vi "Main.vi"() -> ()   [LabVIEW 2022 SP3]
doc: "Use this template to build a simple state machine design pattern. Each state executes code and determines which state to transition to."
uses:
  controls/State.ctl
  <instrlib>/Vision Research Phantom Series Labview Driver/_Type Defs/PHCon IMRANGE.ctl
  <instrlib>/Vision Research Phantom Series Labview Driver/_Type Defs/PhFile InfName.ctl
  <instrlib>/Vision Research Phantom Series Labview Driver/_Type Defs/PhInt PhProcessImage Selectors.ctl
  <instrlib>/Vision Research Phantom Series Labview Driver/_Type Defs/PhInt REDUCE16TO8PARAMS.ctl
  Global 3.vi
  Global 2.vi
  Global 1.vi
  <instrlib>/Vision Research Phantom Series Labview Driver/VRI.lvlib
panel:
  in  "Weave Net":bool
  in  "Step (mm)":dbl=300.0 format="%#_13g"
  in  "Line No 2":i16=100 caption="No. of Rows"
  in  "Row spacing (um)":dbl=100.0 format="%#_13g"
  in  "Direction 2":enum16{"Y to X", "X to Y"}(ring)
  in  "Stall (s)":i16=1
  in  "Row width (mm)":dbl=60.0 format="%#_13g"
  in  "Start Pos":dbl[](array[numeric])=[-30.0, -30.0] caption="Start Point"
  in  "PtP Motion":bool
  out "XY Graph":cluster{"X":dbl, "Y":dbl}[](graph)
  out "Preview":picture
  in  "Stack No":i16=10
  in  "Direction":enum16{"Y to X", "X to Y"}(ring)
  in  "MinJT":dbl=0.02 format="%#_13g"
  in  "MaxJT":dbl=0.02 format="%#_13g"
  in  "Length (mm)":dbl=60.0 format="%#_13g"
  in  "Spacing (um)":dbl=100.0 format="%#_13g"
  in  "Line No":i16=100
  in  "Acc. (mm/s2)":dbl=1500.0 format="%#_13g"
  in  "Vel (mm/s)":dbl=300.0 format="%#_13g"
  in  "Start Point":dbl[](array[numeric])=[-30.0, -30.0]
  in  "OffsetNo":i16=20
  in  "Offsets (um,um)":dbl[](array[numeric])=[100.0, 100.0] format="%#_13g"
  in  "Repeat No":i16=1
  in  "Acc (mm/s2)":dbl=150.0 format="%#_13g"
  in  "Vel (mm/s)":dbl=70.0 format="%#_13g"
  in  "Traj file":string=".trj"
  in  "Start Position":dbl[](array[numeric])=[-30.0, -30.0] format="%#_13g"
  in  "Target":dbl[](array[numeric])=[50.0, -50.0] format="%#_13g"
  in  "Abort Current Motion":bool
  in  "Movement of Parallel Stacking":bool
  in  "Movement of Parallel Wave":bool
  in  "Move to Target":bool
  in  "Move Along Trajectory with an Offset":bool
  in  "Move Along Trajectory":bool
  in  "Disable Stage":bool
  in  "Homing Stage":bool
  in  "Exit":bool
  # "NFES CONTROL PANEL"
  # "Camera Vision"
  # "Needle position monitor"
  # "Move to Target"
  # "Trajectory Motion"
  # "Wave Motion"
  # "Point-to-Point Motion"
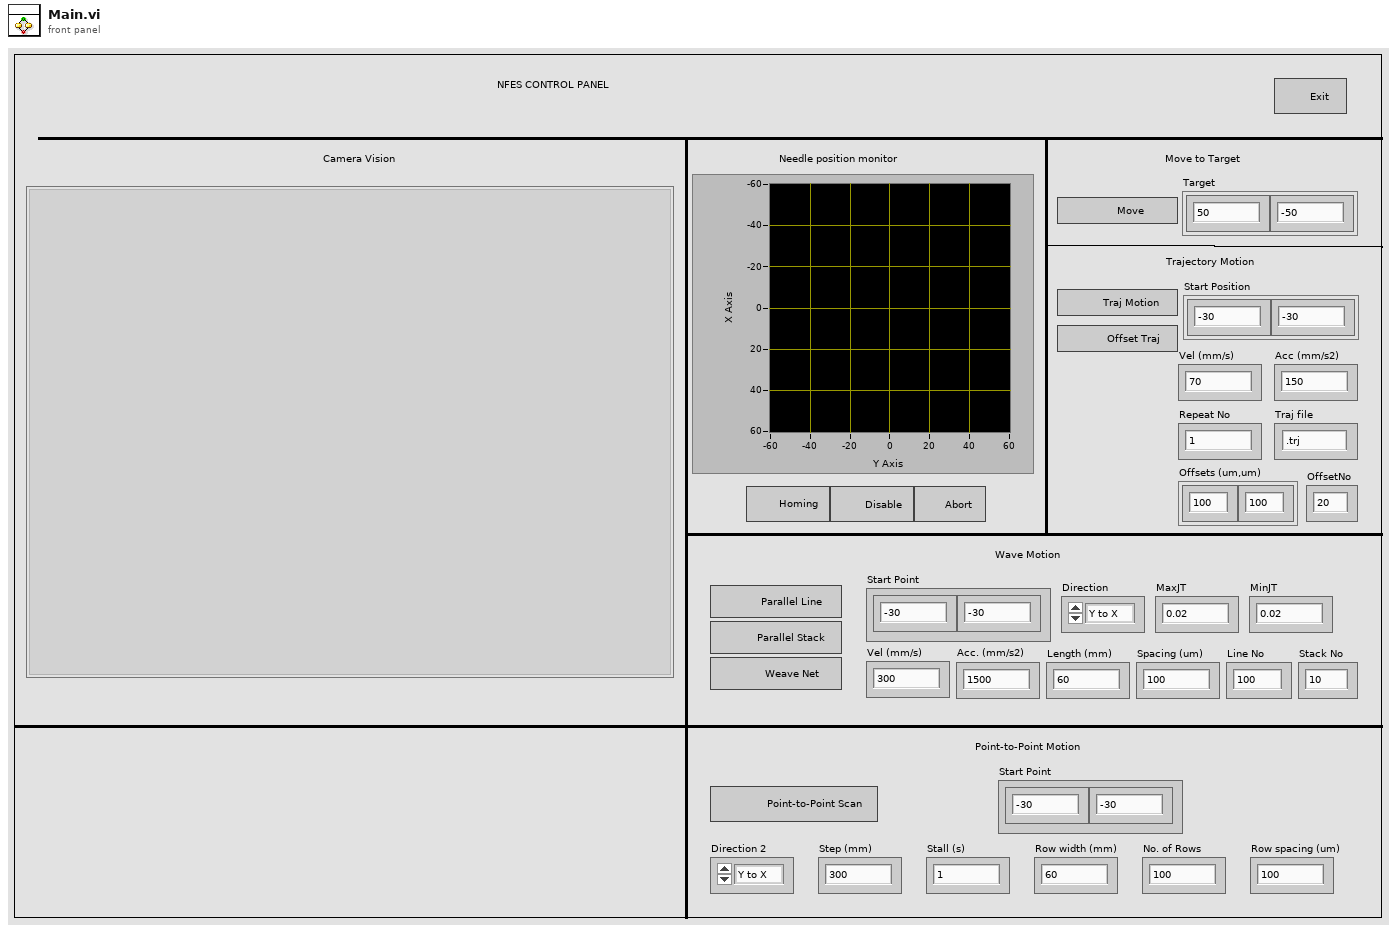
[diagram p1: front panel]
types:
  T1 = typedef "State.ctl" = enum16{"Initialize", "Wait for Event", "Homing", "Disable", "Move", "Trajectory", "Trajoffset", "ParaWave", "ParaStack", "NetWeaving", "PtPMove", "Abort", "Exit"}
  T2 = typedef "VRI.lvlib/PhInt REDUCE16TO8PARAMS.ctl" = cluster{"fGain16_8":dbl}
  T3 = typedef "VRI.lvlib/PhInt PhProcessImage Selectors.ctl" = u16
  T4 = typedef "VRI.lvlib/PhFile InfName.ctl" = u32
  T5 = typedef "VRI.lvlib/PHCon IMRANGE.ctl" = cluster{"First":i32, "Cnt":u32}
  T6 = typedef "VRI.lvlib/PhInt IH.ctl" = cluster{"biSize":u32, "biWidth":i32, "biHeight":i32, "biPlanes":u16, "biBitCount":u16, "biCompresssion":u32, "biSizeImage":u32, "biXPelsPerMeter":i32, "biYPelsPerMeter":i32, "biClrUsed":u32, "biClrImportant":u32, "BlackLevel":i32, "WhiteLevel":i32}
  T7 = typedef "VRI.lvlib/BITMAPINFOHEADER.ctl" = cluster{"biSize":u32, "biWidth":i32, "biHeight":i32, "biPlanes":u16, "biBitCount":u16, "biCompression":u32, "biSizeImage":u32, "biXPelsPerMeter":i32, "biYPelsPerMeter":i32, "biClrUsed":u32, "biClrImportant":u32}
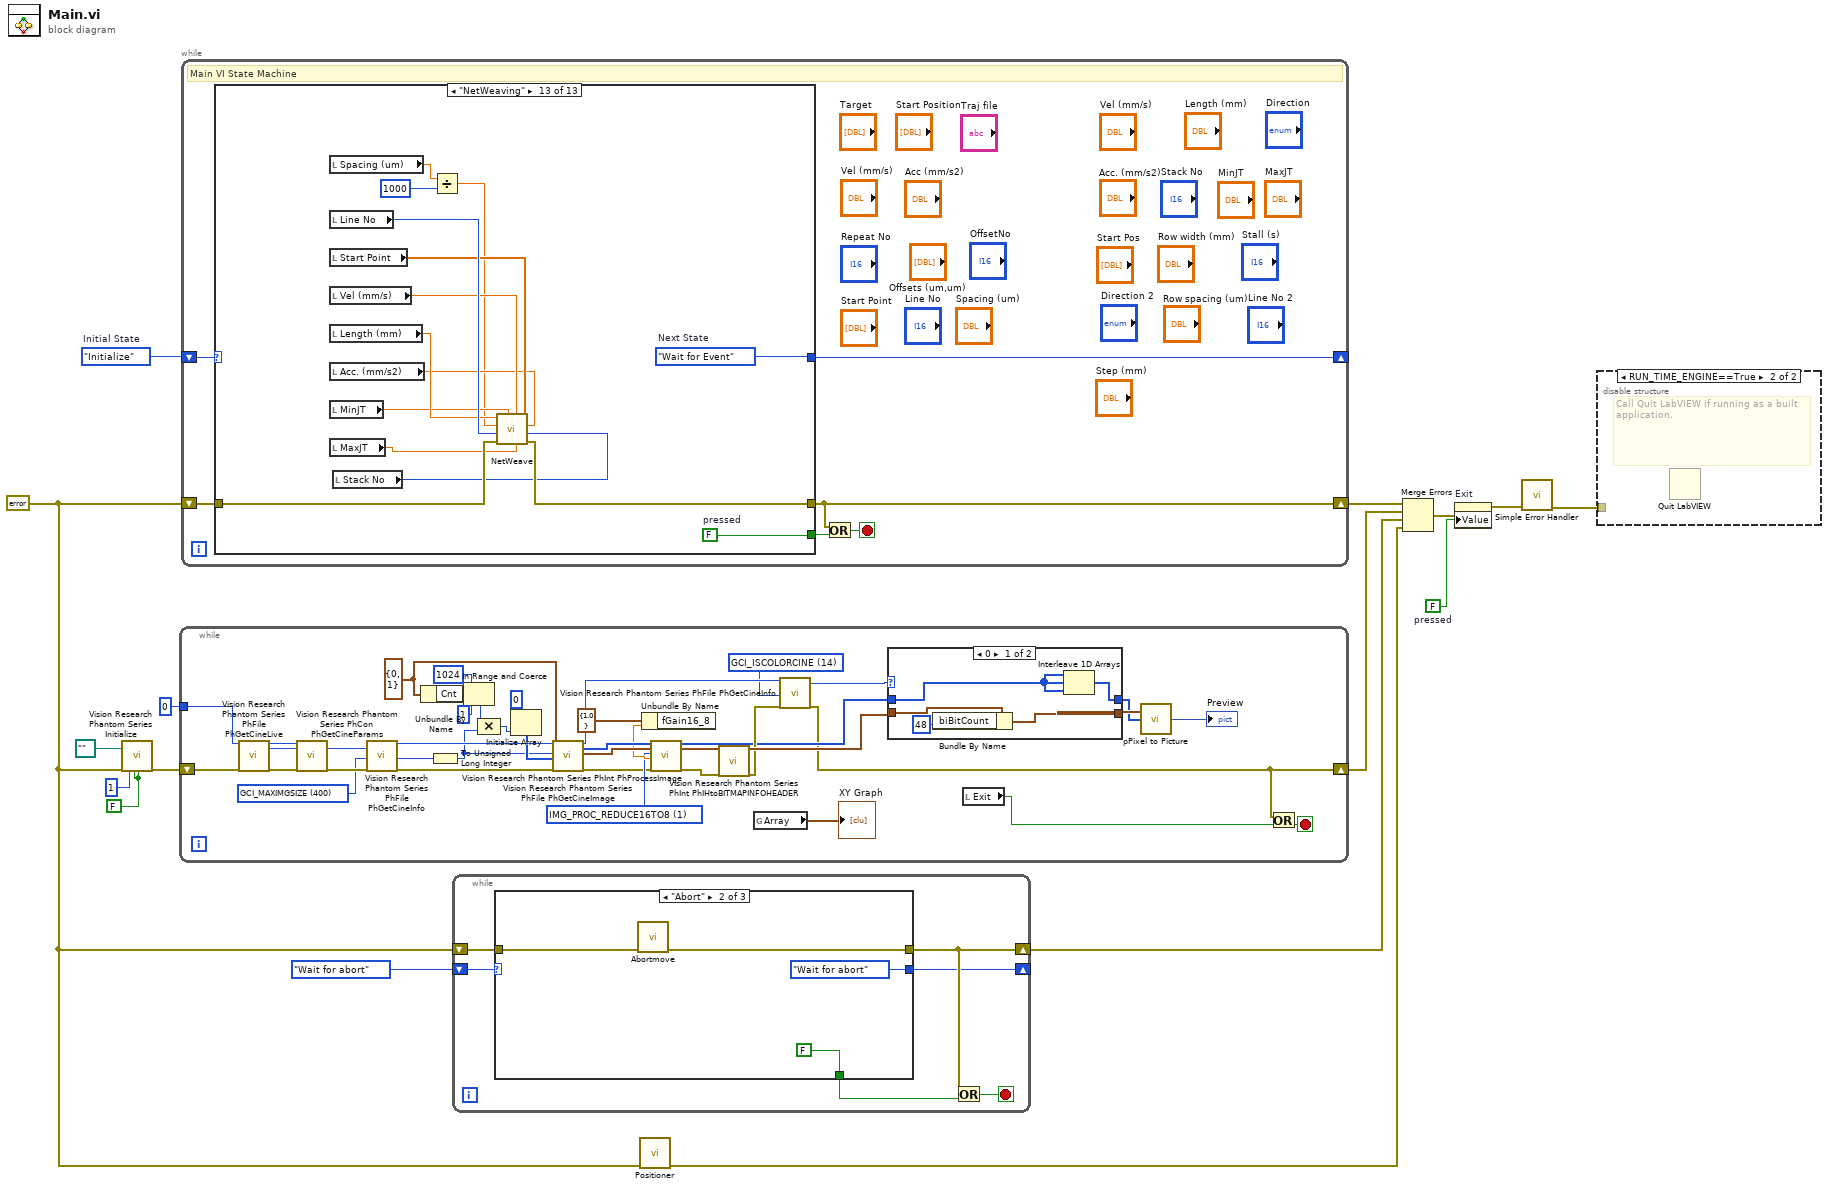
[diagram p0: block diagram]
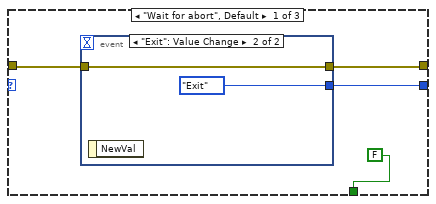
[diagram p2: hidden frame]
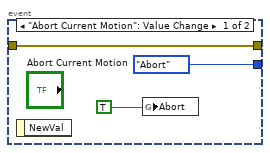
[diagram p3: hidden frame]
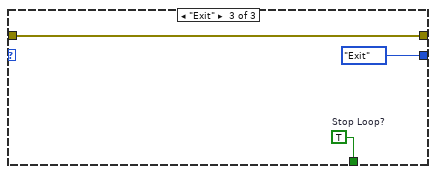
[diagram p4: hidden frame]
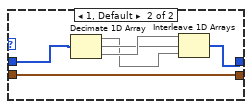
[diagram p5: hidden frame]
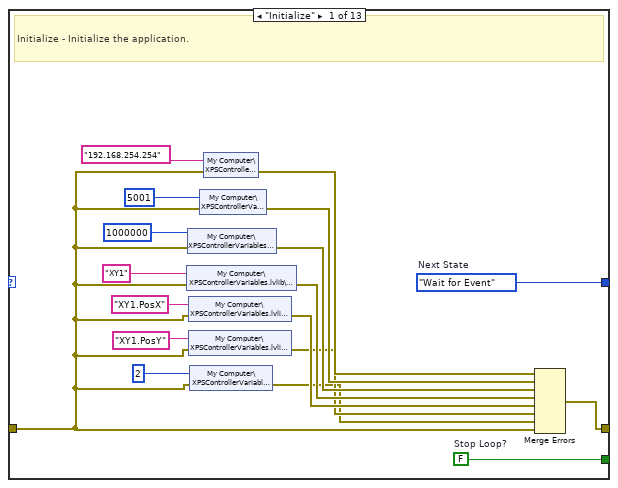
[diagram p7: hidden frame]
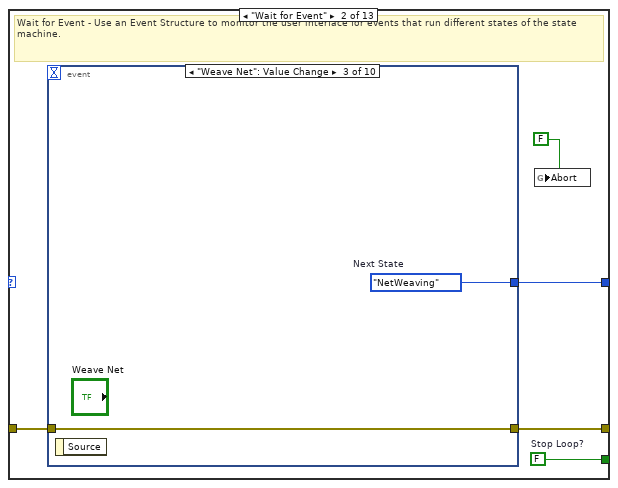
[diagram p8: hidden frame]
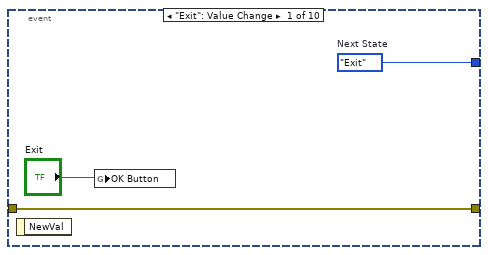
[diagram p9: hidden frame]
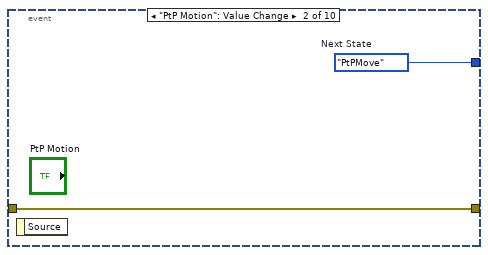
[diagram p10: hidden frame]
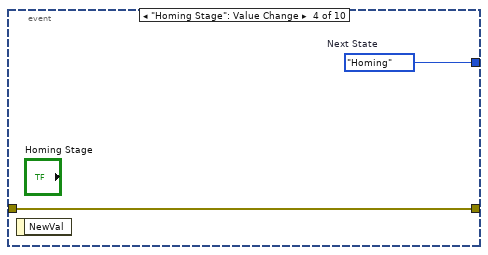
[diagram p11: hidden frame]
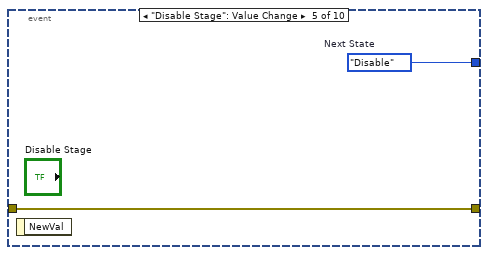
[diagram p12: hidden frame]
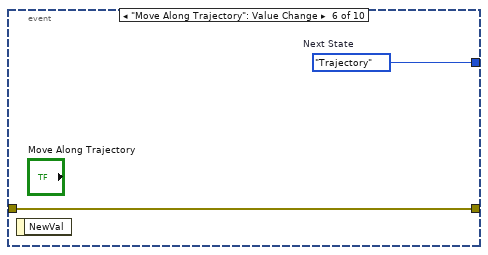
[diagram p13: hidden frame]
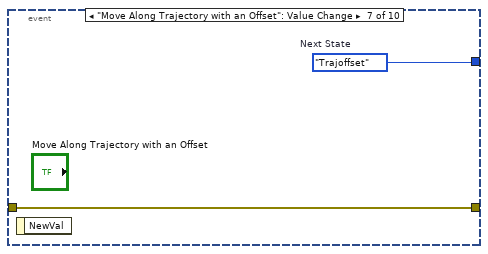
[diagram p14: hidden frame]
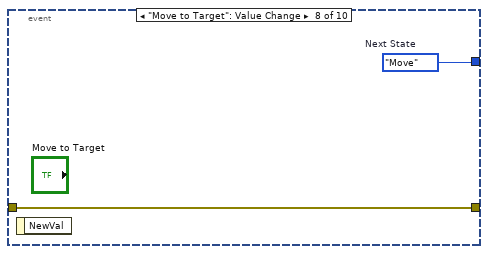
[diagram p15: hidden frame]
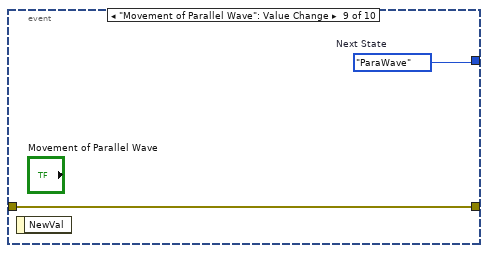
[diagram p16: hidden frame]
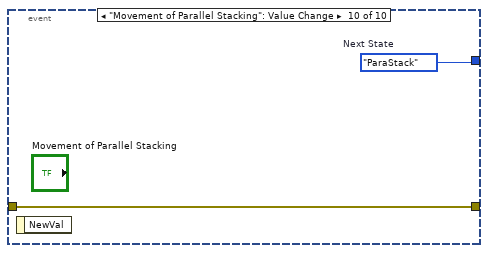
[diagram p17: hidden frame]
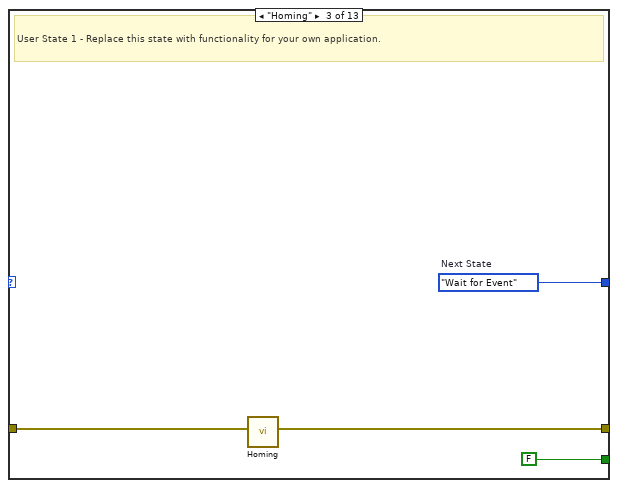
[diagram p18: hidden frame]
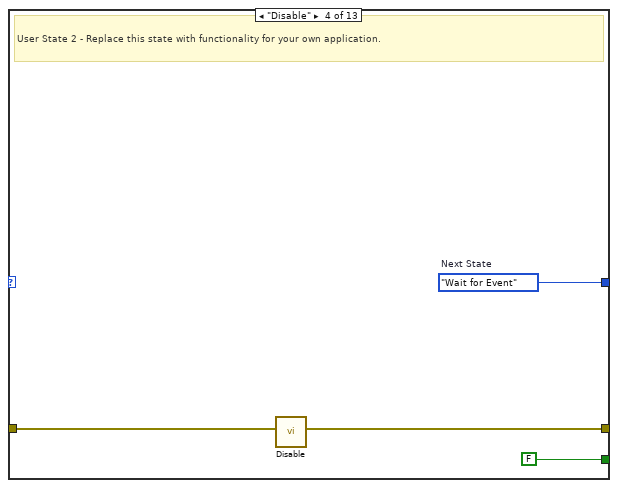
[diagram p19: hidden frame]
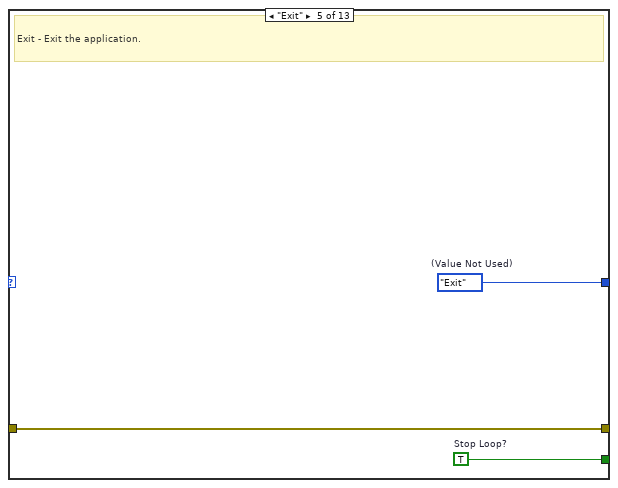
[diagram p20: hidden frame]
diagram:
  w7 = FALSE  # pressed
  w11 = FALSE ("ID Query (T: Check)")
  w2 = errorcluster {"status"=FALSE, "code"=0, "source"=""} ("error constant")
  w16 = State."Initialize"  # Initial State
  n1 = call <instrlib>:"Vision Research Phantom Series Initialize.vi"("Storage Path (\"\")"=path "" ("Storage Path (\"\")"), "error in (no error)"=w2, "CallID"=u32 1, "ID Query (T: Check)"=w11, "Reset (F: Don't Reset)"=w11) -> ("Error Out"=w9:errorcluster)  [unwired: 14 out]
  n2 = while {
    tunnel: u32 0 ("Camera Number") -> [w33]
    shift-right: [w19] -> w8
    shift-left: w9 -> [w31]
    stop <- w20 stop-if-true
    w46 = T3 1 items=["IMG_PROC_REDUCE16TO8"=1] ("procID")
    w21 = T4 14 items=["GCI_CFA"=0, "GCI_FRAMERATE"=1, "GCI_EXPOSURE"=2, "GCI_AUTOEXPOSURE"=3, "GCI_REALBPP"=4, "GCI_CAMERASERIAL"=5, "GCI_HEADSERIAL0"=6, "GCI_HEADSERIAL1"=7, "GCI_HEADSERIAL2"=8, "GCI_HEADSERIAL3"=9, "GCI_TRIGTIMESEC"=10, "GCI_TRIGTIMEFR"=11, "GCI_ISFILECINE"=12, "GCI_IS16BPPCINE"=13, "GCI_ISCOLORCINE"=14, "GCI_ISMULTIHEADCINE"=15, "GCI_EXPOSURENS"=16, "GCI_EDREXPOSURENS"=17, "GCI_FRAMEDELAYNS"=19, "GCI_FROMFILETYPE"=20, "GCI_COMPRESSION"=21, "GCI_CAMERAVERSION"=22, "GCI_ROTATE"=23, "GCI_IMWIDTH"=24, "GCI_IMHEIGHT"=25, "GCI_IMWIDTHACQ"=26, "GCI_IMHEIGHTACQ"=27, "GCI_POSTTRIGGER"=28, "GCI_IMAGECOUNT"=29, "GCI_TOTALIMAGECOUNT"=30, "GCI_TRIGFRAME"=31, "GCI_AUTOEXPLEVEL"=32, "GCI_AUTOEXPTOP"=33, "GCI_AUTOEXPLEFT"=34, "GCI_AUTOEXPBOTTOM"=35, "GCI_AUTOEXPRIGHT"=36, "GCI_RECORDINGTIMEZONE"=37, "GCI_FIRSTIMAGENO"=38, "GCI_FIRSTMOVIEIMAGE"=39, "GCI_CINENAME"=40, "GCI_FRPSTEPS"=100, "GCI_FRP1X"=101, "GCI_FRP1Y"=102, "GCI_FRP2X"=103, "GCI_FRP2Y"=104, "GCI_FRP3X"=105, "GCI_FRP3Y"=106, "GCI_FRP4X"=107, "GCI_FRP4Y"=108, "GCI_WRITEERR"=109, "GCI_LENSDESCRIPTION"=110, "GCI_LENSAPERATURE"=111, "GCI_LENSFOCALLENGTH"=112, "GCI_WB"=200, "GCI_WBVIEW"=201, "GCI_BRIGHT"=202, "GCI_CONTRAST"=203, "GCI_GAMMA"=204, "GCI_GAMMAR"=223, "GCI_GAMMAB"=224, "GCI_SATURATION"=205, "GCI_HUE"=206, "GCI_FLIPH"=207, "GCI_FLIPV"=208, "GCI_FILTERCODE"=209, "GCI_IMFILTER"=210, "GCI_INTALGO"=211, "GCI_PEDESTALR"=212, "GCI_PEDESTALG"=213, "GCI_PEDESTALB"=214, "GCI_FLARE"=225, "GCI_CHROMA"=226, "GCI_TONE"=227, "GCI_ENABLEMATRICES"=228, "GCI_USERMATRIX"=229, "GCI_RESAMPLEACTIVE"=215, "GCI_RESAMPLEWIDTH"=216, "GCI_RESAMPLEHEIGHT"=217, "GCI_CROPACTIVE"=218, "GCI_CROPRECTANGLE"=219, "GCI_OFFSET16_8"=220, "GCI_GAIN16_8"=221, "GCI_DEMOSAICINGFUNCPTR"=222, "GCI_VFLIPVIEWACTIVE"=300, "GCI_MAXIMGSIZE"=400, "GCI_FRPIMGNOARRAY"=450, "GCI_FRPRATEARRAY"=451, "GCI_FRPSHAPEARRAY"=452, "GCI_TRIGTC"=470, "GCI_TRIGTCU"=471, "GCI_PBRATE"=472, "GCI_TCRATE"=473, "GCI_SAVERANGE"=500, "GCI_SAVEFILENAME"=501, "GCI_SAVEFILETYPE"=502, "GCI_SAVE16BIT"=503, "GCI_SAVEPACKED"=504, "GCI_SAVEXML"=505, "GCI_SAVESTAMPTIME"=506, "GCI_SAVEAVIFRAMERATE"=520, "GCI_SAVEAVICOMPRESSORLIST"=521, "GCI_SAVEAVICOMPRESSORINDEX"=522, "GCI_SAVEDPXLSB"=530, "GCI_SAVEDPXTO10BPS"=531, "GCI_SAVEDPXDATAPACKING"=532, "GCI_SAVEDPX10BITLOG"=533, "GCI_SAVEDPXEXPORTLOGLUT"=534, "GCI_SAVEDPX10BITLOGREFWHITE"=535, "GCI_SAVEDPX10BITLOGREFBLACK"=536, "GCI_SAVEDPX10BITLOGGAMMA"=537, "GCI_SAVEDPX10BITLOGFILMGAMMA"=538, "GCI_SAVEQTPLAYBACKRATE"=550, "GCI_SAVECCIQUALITY"=560, "GCI_UNCALIBRATEDIMAGE"=600, "GCI_NOPROCESSING"=601, "GCI_BADPIXELREPAIR"=602] ("InfName")
    w32 = T4 400 items=["GCI_CFA"=0, "GCI_FRAMERATE"=1, "GCI_EXPOSURE"=2, "GCI_AUTOEXPOSURE"=3, "GCI_REALBPP"=4, "GCI_CAMERASERIAL"=5, "GCI_HEADSERIAL0"=6, "GCI_HEADSERIAL1"=7, "GCI_HEADSERIAL2"=8, "GCI_HEADSERIAL3"=9, "GCI_TRIGTIMESEC"=10, "GCI_TRIGTIMEFR"=11, "GCI_ISFILECINE"=12, "GCI_IS16BPPCINE"=13, "GCI_ISCOLORCINE"=14, "GCI_ISMULTIHEADCINE"=15, "GCI_EXPOSURENS"=16, "GCI_EDREXPOSURENS"=17, "GCI_FRAMEDELAYNS"=19, "GCI_FROMFILETYPE"=20, "GCI_COMPRESSION"=21, "GCI_CAMERAVERSION"=22, "GCI_ROTATE"=23, "GCI_IMWIDTH"=24, "GCI_IMHEIGHT"=25, "GCI_IMWIDTHACQ"=26, "GCI_IMHEIGHTACQ"=27, "GCI_POSTTRIGGER"=28, "GCI_IMAGECOUNT"=29, "GCI_TOTALIMAGECOUNT"=30, "GCI_TRIGFRAME"=31, "GCI_AUTOEXPLEVEL"=32, "GCI_AUTOEXPTOP"=33, "GCI_AUTOEXPLEFT"=34, "GCI_AUTOEXPBOTTOM"=35, "GCI_AUTOEXPRIGHT"=36, "GCI_RECORDINGTIMEZONE"=37, "GCI_FIRSTIMAGENO"=38, "GCI_FIRSTMOVIEIMAGE"=39, "GCI_CINENAME"=40, "GCI_FRPSTEPS"=100, "GCI_FRP1X"=101, "GCI_FRP1Y"=102, "GCI_FRP2X"=103, "GCI_FRP2Y"=104, "GCI_FRP3X"=105, "GCI_FRP3Y"=106, "GCI_FRP4X"=107, "GCI_FRP4Y"=108, "GCI_WRITEERR"=109, "GCI_LENSDESCRIPTION"=110, "GCI_LENSAPERATURE"=111, "GCI_LENSFOCALLENGTH"=112, "GCI_WB"=200, "GCI_WBVIEW"=201, "GCI_BRIGHT"=202, "GCI_CONTRAST"=203, "GCI_GAMMA"=204, "GCI_GAMMAR"=223, "GCI_GAMMAB"=224, "GCI_SATURATION"=205, "GCI_HUE"=206, "GCI_FLIPH"=207, "GCI_FLIPV"=208, "GCI_FILTERCODE"=209, "GCI_IMFILTER"=210, "GCI_INTALGO"=211, "GCI_PEDESTALR"=212, "GCI_PEDESTALG"=213, "GCI_PEDESTALB"=214, "GCI_FLARE"=225, "GCI_CHROMA"=226, "GCI_TONE"=227, "GCI_ENABLEMATRICES"=228, "GCI_USERMATRIX"=229, "GCI_RESAMPLEACTIVE"=215, "GCI_RESAMPLEWIDTH"=216, "GCI_RESAMPLEHEIGHT"=217, "GCI_CROPACTIVE"=218, "GCI_CROPRECTANGLE"=219, "GCI_OFFSET16_8"=220, "GCI_GAIN16_8"=221, "GCI_DEMOSAICINGFUNCPTR"=222, "GCI_VFLIPVIEWACTIVE"=300, "GCI_MAXIMGSIZE"=400, "GCI_FRPIMGNOARRAY"=450, "GCI_FRPRATEARRAY"=451, "GCI_FRPSHAPEARRAY"=452, "GCI_TRIGTC"=470, "GCI_TRIGTCU"=471, "GCI_PBRATE"=472, "GCI_TCRATE"=473, "GCI_SAVERANGE"=500, "GCI_SAVEFILENAME"=501, "GCI_SAVEFILETYPE"=502, "GCI_SAVE16BIT"=503, "GCI_SAVEPACKED"=504, "GCI_SAVEXML"=505, "GCI_SAVESTAMPTIME"=506, "GCI_SAVEAVIFRAMERATE"=520, "GCI_SAVEAVICOMPRESSORLIST"=521, "GCI_SAVEAVICOMPRESSORINDEX"=522, "GCI_SAVEDPXLSB"=530, "GCI_SAVEDPXTO10BPS"=531, "GCI_SAVEDPXDATAPACKING"=532, "GCI_SAVEDPX10BITLOG"=533, "GCI_SAVEDPXEXPORTLOGLUT"=534, "GCI_SAVEDPX10BITLOGREFWHITE"=535, "GCI_SAVEDPX10BITLOGREFBLACK"=536, "GCI_SAVEDPX10BITLOGGAMMA"=537, "GCI_SAVEDPX10BITLOGFILMGAMMA"=538, "GCI_SAVEQTPLAYBACKRATE"=550, "GCI_SAVECCIQUALITY"=560, "GCI_UNCALIBRATEDIMAGE"=600, "GCI_NOPROCESSING"=601, "GCI_BADPIXELREPAIR"=602] ("InfName")
    w34 = T5 {"First"=0, "Cnt"=1} ("pRng")
    n3 = call <instrlib>:"Vision Research Phantom Series PhFile PhGetCineLive.vi"("CN (in)"=w33, "Error In (no error)"=w31) -> ("CN (out)"=w40:u32, "pCH (out)"=w54:u64, "Error Out"=w42:errorcluster)  [unwired: 15 in]
    n4 = call <instrlib>:"Vision Research Phantom Series PhCon PhGetCineParams.vi"("CN in"=w40, "Error In (no error)"=w42) -> ("Error Out"=w41:errorcluster)  [unwired: 1 in, 16 out]
    n5 = call <instrlib>:"Vision Research Phantom Series PhFile PhGetCineInfo.vi"("CH in"=w54, "InfName"=w32, "Error In (no error)"=w41) -> ("CH out"=w52:u64, "pInfVal out"=w25:i32, "Error Out"=w50:errorcluster)  [unwired: 14 in]
    n6 = Unbundle By Name(w34) -> ("Cnt"=w39:u32)
    n7 = To Unsigned Long Integer(number=w25) -> (unsigned 32bit integer=w24:u32)
    n8 = In Range and Coerce(upper limit=u32 1024, x=w39, lower limit=u32 1) -> (coerced(x)=w38:u32)  [unwired: 1 out]
    n9 = Compound Arithmetic op=MULTIPLY(w38, w24) -> (w35:u32)
    n10 = Initialize Array(u16 0 ("element"), w35) -> (w51:u16[])
    n11 = call <instrlib>:"Vision Research Phantom Series PhFile PhGetCineImage.vi"("hC [in]"=w52, "pRng [in]"=w34, "bufferByteSize [in]"=w24, "pPixelBuffer [in]"=w51, "Error In (no error)"=w50) -> ("hC [out]"=w30:u64, "pPixelBuffer [out]"=w49:u16[], "IH [out]"=w48:T6, "Error Out"=w45:errorcluster)  [unwired: 11 in]
    n12 = Unbundle By Name(T2 {"fGain16_8"=1.0} ("REDUCE16TO8PARAMS")) -> ("fGain16_8"=w47:dbl)
    n13 = call <instrlib>:"Vision Research Phantom Series PhInt PhProcessImage.vi"("pPixelSrc [in]"=w49, "IH [in]"=w48, "procID"=w46, "pProcParams"=w47, "Error In (no error)"=w45) -> ("pPixelDest [out]"=w22:u8[], "IH [out]"=w43:T6, "Error Out"=w44:errorcluster)  [unwired: 12 in]
    n14 = call <instrlib>:"Vision Research Phantom Series PhInt PhIHtoBITMAPINFOHEADER.vi"("IH"=w43, "Error In (no error)"=w44) -> ("BITMAPINFOHEADER"=w28:T7, "Error Out"=w26:errorcluster)  [unwired: 16 in]
    n15 = global read "Global 1.vi" "Array"() -> (→"XY Graph":cluster{"Numeric":dbl, "Numeric 2":dbl}[])
    n16 = call <instrlib>:"Vision Research Phantom Series PhFile PhGetCineInfo.vi"("CH in"=w30, "InfName"=w21, "Error In (no error)"=w26) -> ("pInfVal out"=w29:i32, "Error Out"=w19:errorcluster)  [unwired: 14 in, 1 out]
    n17 = case shown="0" w29 {
      tunnel: [w58 w62] -> w23
      tunnel: w28 -> [w61 w67]
      tunnel: [w60 w67] -> w27
      tunnel: w22 -> [w57 w63]
      frame 0 {
        n18 = Bundle By Name(cluster=w61, "biBitCount"=u16 48) -> (w60:T7)
        n19 = Interleave 1D Arrays(w57, w57, w57) -> (w58:u8[])
      }
      frame 1, Default {
        n20 = Decimate 1D Array(w63) -> (w64:u8[], w65:u8[], w66:u8[])
        n21 = Interleave 1D Arrays(w66, w65, w64) -> (w62:u8[])
      }
    }
    n22 = local read "Exit"() -> (w18:bool)
    n23 = call <instrlib>:"pPixel to Picture.vi"("pPixel"=w23, "BITMAPINFOHEADER"=w27) -> ("Preview"=→"Preview":picture)  [unwired: 1 in]
    n24 = Or(x=w19, y=w18) -> (x .or. y?=w20:bool)
  }
  n25 = while {
    shift-right: [w72] -> _
    shift-left: w16 -> [w73]
    shift-right: [w68] -> w14
    shift-left: w2 -> [w71]
    stop <- w69 stop-if-true
    # "Main VI State Machine"
    n26 = case shown="\"NetWeaving\"" w73 {
      tunnel: [w91 w96 w121 w125 w128 w131 w142 w155 w170 w186 w188 w193 w207] -> w72
      tunnel: [w90 w95 FALSE ("Stop Loop?") FALSE ("Stop Loop?") w127 FALSE ("Stop Loop?") FALSE ("Stop Loop?") FALSE ("Stop Loop?") FALSE ("Stop Loop?") FALSE ("Stop Loop?") FALSE ("Stop Loop?") FALSE ("Stop Loop?") w216] -> w70
      tunnel: w71 -> [w75 w94 w119 w123 w126 w133 w140 w153 w168 w184 w189 w203 w218]
      tunnel: [w74 w93 w118 w122 w126 w132 w139 w152 w167 w183 w189 w202 w217] -> w68
      frame "Initialize" {
        w90 = FALSE  # Stop Loop?
        w91 = State."Wait for Event"  # Next State
        # "Initialize - Initialize the application."
        n27 = shared-variable "My Computer\\XPSControllerVariables.lvlib\\GroupName"("XY1", error in=w75) -> (error out=w79:errorcluster)
        n28 = shared-variable "My Computer\\XPSControllerVariables.lvlib\\Timeout"(1000000, error in=w75) -> (error out=w80:errorcluster)
        n29 = shared-variable "My Computer\\XPSControllerVariables.lvlib\\PosNameX"("XY1.PosX", error in=w75) -> (error out=w78:errorcluster)
        n30 = shared-variable "My Computer\\XPSControllerVariables.lvlib\\PosNameY"("XY1.PosY", error in=w75) -> (error out=w77:errorcluster)
        n31 = shared-variable "My Computer\\XPSControllerVariables.lvlib\\nbitem"(2, error in=w75) -> (error out=w76:errorcluster)
        n32 = shared-variable "My Computer\\XPSControllerVariables.lvlib\\Port"(5001, error in=w75) -> (error out=w81:errorcluster)
        n33 = shared-variable "My Computer\\XPSControllerVariables.lvlib\\IP"("192.168.254.254", error in=w75) -> (error out=w82:errorcluster)
        n34 = Merge Errors(w82, w81, w80, w79, w78, w77, w76, w75) -> (w74:errorcluster)
      }
      frame "Wait for Event" {
        w95 = FALSE  # Stop Loop?
        # "Wait for Event - Use an Event Structure to monitor the user interface for events that run different states of the state machine."
        n35 = event shown="[2] \"Weave Net\": Value Change" {
          selector: _ -> [_ _ _ _ _ _ _ _ _ _]
          dyn-events: _ -> [_ _ _ _ _ _ _ _ _ _]
          timeout: _ -> [_ _ _ _ _ _ _ _ _ _]
          tunnel: [w99 w100 w102 w105 w107 w108 w110 w112 w114 w116] -> w96
          tunnel: w94 -> [w98 w101 w103 w104 w106 w109 w111 w113 w115 w117]
          tunnel: [w98 w101 w103 w104 w106 w109 w111 w113 w115 w117] -> w93
          event "Exit": Value Change {
            w99 = State."Exit"  # Next State
            n36 = event-data() -> ()  [unwired: 1 in, 1 out]
            n37 = global write "Global 2.vi" "OK Button"("Exit") -> ()
          }
          event "PtP Motion": Value Change {
            w100 = State."PtPMove"  # Next State
            n38 = event-data() -> ()  [unwired: 1 in, 1 out]
          }
          event "Weave Net": Value Change {
            w102 = State."NetWeaving"  # Next State
            n39 = event-data() -> ()  [unwired: 1 in, 1 out]
          }
          event "Homing Stage": Value Change {
            w105 = State."Homing"  # Next State
            n40 = event-data() -> ()  [unwired: 1 in, 1 out]
          }
          event "Disable Stage": Value Change {
            w107 = State."Disable"  # Next State
            n41 = event-data() -> ()  [unwired: 1 in, 1 out]
          }
          event "Move Along Trajectory": Value Change {
            w108 = State."Trajectory"  # Next State
            n42 = event-data() -> ()  [unwired: 1 in, 1 out]
          }
          event "Move Along Trajectory with an Offset": Value Change {
            w110 = State."Trajoffset"  # Next State
            n43 = event-data() -> ()  [unwired: 1 in, 1 out]
          }
          event "Move to Target": Value Change {
            w112 = State."Move"  # Next State
            n44 = event-data() -> ()  [unwired: 1 in, 1 out]
          }
          event "Movement of Parallel Wave": Value Change {
            w114 = State."ParaWave"  # Next State
            n45 = event-data() -> ()  [unwired: 1 in, 1 out]
          }
          event "Movement of Parallel Stacking": Value Change {
            w116 = State."ParaStack"  # Next State
            n46 = event-data() -> ()  [unwired: 1 in, 1 out]
          }
        }
        n47 = global write "Global 3.vi" "Abort"(FALSE ("Stop Loop?")) -> ()
      }
      frame "Homing" {
        w121 = State."Wait for Event"  # Next State
        # "User State 1 - Replace this state with functionality for your own application."
        n48 = call "Homing.vi"("error in"=w119) -> ("error out"=w118:errorcluster)  [unwired: 10 in]
      }
      frame "Disable" {
        w125 = State."Wait for Event"  # Next State
        # "User State 2 - Replace this state with functionality for your own application."
        n49 = call "Disable.vi"("error in"=w123) -> ("error out"=w122:errorcluster)  [unwired: 10 in]
      }
      frame "Exit" {
        w127 = TRUE  # Stop Loop?
        w128 = State."Exit"  # (Value Not Used)
        # "Exit - Exit the application."
      }
      frame "Move" {
        w131 = State."Wait for Event"  # Next State
        n50 = local read "Target"() -> (w129:dbl[])
        n51 = call "AbsMove.vi"("Pos"=w129, "error in"=w133) -> ("error out"=w132:errorcluster)  [unwired: 9 in]
      }
      frame "Trajectory" {
        w142 = State."Wait for Event"  # Next State
        n52 = local read "Traj file"() -> (w137:string)
        n53 = local read "Start Position"() -> (w138:dbl[])
        n54 = local read "Repeat No"() -> (w134:i16)
        n55 = local read "Vel (mm/s)"() -> (w136:dbl)
        n56 = local read "Acc (mm/s2)"() -> (w135:dbl)
        n57 = call "Traj.vi"("error in"=w140, "StartPos"=w138, "Repeat number"=w134, "Acc"=w135, "Vel"=w136, "String"=w137) -> ("error out"=w139:errorcluster)  [unwired: 5 in]
      }
      frame "Trajoffset" {
        w155 = State."Wait for Event"  # Next State
        n58 = local read "Offsets (um,um)"() -> (w145:dbl[])
        n59 = local read "Traj file"() -> (w150:string)
        n60 = local read "Repeat No"() -> (w149:i16)
        n61 = local read "Start Position"() -> (w151:dbl[])
        n62 = local read "OffsetNo"() -> (w146:i16)
        n63 = local read "Vel (mm/s)"() -> (w148:dbl)
        n64 = local read "Acc (mm/s2)"() -> (w147:dbl)
        n65 = Divide(x=w145, y=1000) -> (x/y=w143:dbl[])
        n66 = call "TrajOffset.vi"("OffsetNo"=w146, "Offsets"=w143, "StartPos"=w151, "Repeat number"=w149, "error in"=w153, "Acc"=w147, "Vel"=w148, "FileName"=w150) -> ("error out"=w152:errorcluster)  [unwired: 3 in]
      }
      frame "ParaWave" {
        w170 = State."Wait for Event"  # Next State
        n67 = local read "Start Point"() -> (w162:dbl[])
        n68 = local read "MinJT"() -> (w161:dbl)
        n69 = local read "Length (mm)"() -> (w166:dbl)
        n70 = local read "Spacing (um)"() -> (w158:dbl)
        n71 = local read "Line No"() -> (w165:i16)
        n72 = local read "MaxJT"() -> (w160:dbl)
        n73 = local read "Vel (mm/s)"() -> (w163:dbl)
        n74 = local read "Acc. (mm/s2)"() -> (w164:dbl)
        n75 = Divide(x=w158, y=1000) -> (x/y=w156:dbl)
        n76 = local read "Direction"() -> (w159:enum16{"Y to X", "X to Y"})
        n77 = call "WaveMove.vi"("Length"=w166, "Spacing"=w156, "LineNo"=w165, "error in"=w168, "MinJT"=w161, "Vel"=w163, "MaxJT"=w160, "StartPos"=w162, "Acc"=w164, "Direction"=w159) -> ("error out"=w167:errorcluster)
      }
      frame "ParaStack" {
        w186 = State."Wait for Event"  # Next State
        n78 = local read "Line No"() -> (w182:i16)
        n79 = local read "Direction"() -> (w180:enum16{"Y to X", "X to Y"})
        n80 = local read "Start Point"() -> (w181:dbl[])
        n81 = local read "Length (mm)"() -> (w176:dbl)
        n82 = local read "Stack No"() -> (w174:i16)
        n83 = local read "Spacing (um)"() -> (w172:dbl)
        n84 = local read "Vel (mm/s)"() -> (w175:dbl)
        n85 = local read "Acc. (mm/s2)"() -> (w177:dbl)
        n86 = Divide(x=w172, y=1000) -> (x/y=w171:dbl)
        n87 = local read "MinJT"() -> (w178:dbl)
        n88 = local read "MaxJT"() -> (w179:dbl)
        n89 = call "ParaStack.vi"("StartPos"=w181, "Direction"=w180, "LineNo"=w182, "MinJT"=w178, "Vel"=w175, "MaxJT"=w179, "Length"=w176, "Acc"=w177, "error in"=w184, "StackNo"=w174, "Spacing"=w171) -> ("error out"=w183:errorcluster)  [unwired: 4 in]
      }
      frame "Abort" {
        w188 = State."Wait for Event"  # Next State
      }
      frame "PtPMove" {
        w193 = State."Wait for Event"  # Next State
        w191 = 1000
        n90 = local read "Step (mm)"() -> (w201:dbl)
        n91 = local read "Line No 2"() -> (w200:i16)
        n92 = local read "Row spacing (um)"() -> (w192:dbl)
        n93 = local read "Direction 2"() -> (w199:enum16{"Y to X", "X to Y"})
        n94 = local read "Stall (s)"() -> (w195:i16)
        n95 = local read "Row width (mm)"() -> (w198:dbl)
        n96 = local read "Start Pos"() -> (w197:dbl[])
        n97 = Multiply(x=w195, y=w191) -> (x*y=w196:i32)
        n98 = Divide(x=w192, y=w191) -> (x/y=w190:dbl)
        n99 = call "PtoP.vi"("Spacing"=w190, "LineNo"=w200, "Direction"=w199, "Step"=w201, "error in"=w203, "Wait time"=w196, "Length"=w198, "StartPos"=w197) -> ("error out"=w202:errorcluster)  [unwired: 3 in]
      }
      frame "NetWeaving" {
        w207 = State."Wait for Event"  # Next State
        w216 = FALSE  # pressed
        n100 = local read "Spacing (um)"() -> (w205:dbl)
        n101 = local read "Line No"() -> (w215:i16)
        n102 = local read "Start Point"() -> (w214:dbl[])
        n103 = local read "Vel (mm/s)"() -> (w213:dbl)
        n104 = local read "Length (mm)"() -> (w212:dbl)
        n105 = local read "Acc. (mm/s2)"() -> (w211:dbl)
        n106 = local read "MinJT"() -> (w210:dbl)
        n107 = local read "MaxJT"() -> (w209:dbl)
        n108 = local read "Stack No"() -> (w208:i16)
        n109 = Divide(x=w205, y=1000) -> (x/y=w204:dbl)
        n110 = call "NetWeave.vi"("Length"=w212, "Spacing"=w204, "LineNo"=w215, "error in"=w218, "MinJT"=w210, "Vel"=w213, "MaxJT"=w209, "StartPos"=w214, "Acc"=w211, "LayerNo"=w208) -> ("error out"=w217:errorcluster)
      }
    }
    n111 = Or(x=w68, y=w70) -> (x .or. y?=w69:bool)
  }
  n112 = while {
    shift-right: [w221] -> w4
    shift-left: w2 -> [w224]
    shift-right: [w220] -> _
    shift-left: enum16{"Wait for abort", "Abort", "Exit"}."Wait for abort" -> [w222]
    stop <- w223 stop-if-true
    n113 = case shown="\"Abort\"" w222 {
      tunnel: w224 -> [w227 w237 w240]
      tunnel: [w228 w236 w240] -> w221
      tunnel: [w226 enum16{"Wait for abort", "Abort", "Exit"}."Wait for abort" enum16{"Wait for abort", "Abort", "Exit"}."Exit"] -> w220
      tunnel: [FALSE ("Stop Loop?") FALSE ("Stop Loop?") w238] -> w219
      frame "Wait for abort", Default {
        n114 = event shown="[1] \"Exit\": Value Change" {
          selector: _ -> [_ _]
          dyn-events: _ -> [_ _]
          timeout: _ -> [_ _]
          tunnel: [w230 w233] -> w228
          tunnel: w227 -> [w230 w233]
          tunnel: [enum16{"Wait for abort", "Abort", "Exit"}."Abort" enum16{"Wait for abort", "Abort", "Exit"}."Exit"] -> w226
          event "Abort Current Motion": Value Change {
            n115 = event-data() -> ()  [unwired: 1 in, 1 out]
            n116 = global write "Global 3.vi" "Abort"(TRUE ("Stop Loop?")) -> ()
          }
          event "Exit": Value Change {
            n117 = event-data() -> ()  [unwired: 1 in, 1 out]
          }
        }
      }
      frame "Abort" {
        n118 = call "Abortmove.vi"("error in"=w237) -> ("error out"=w236:errorcluster)  [unwired: 10 in]
      }
      frame "Exit" {
        w238 = TRUE  # Stop Loop?
      }
    }
    n119 = Or(x=w221, y=w219) -> (x .or. y?=w223:bool)
  }
  n120 = call "Positioner.vi"("error in"=w2) -> ("error out"=w1:errorcluster)  [unwired: 10 in]
  n121 = Merge Errors(w14, w8, w4, w1) -> (w6:errorcluster)
  n122 = property on="Exit" class="Bool (strict)"(error in=w6, "Value"=w7) -> (error out=w5:errorcluster)  [unwired: 1 in, 1 out]
  n123 = call <vilib>:"Simple Error Handler.vi"("error in (no error)"=w5) -> ("error out"=w15:errorcluster)  [unwired: 4 in, 4 out]
  n124 = disable-structure shown="RUN_TIME_ENGINE==True" {
    disable-tunnel: w15 -> [_ _]
    frame condition #0 (active) {
    }
    frame condition #1 {
      # "Call Quit LabVIEW if running as a built application."
      n125 = Quit LabVIEW() -> ()  [unwired: 1 in]
    }
  }
